vi "Command & Ack - Destroy Endpoints.vi"(8 "error in (no error)":errorcluster, 11 "SV B-M (Target) in":refnum<class "SV B-M (Target).lvclass">) -> (0 "error out":errorcluster, 3 "SV B-M (Target) out":refnum<class "SV B-M (Target).lvclass">)   [LabVIEW 2015, in "SV B-M (Target).lvclass"]
uses:
  SV B-M (Target).lvclass
  SV B-M (Target).lvclass/SV B-M (Target).ctl
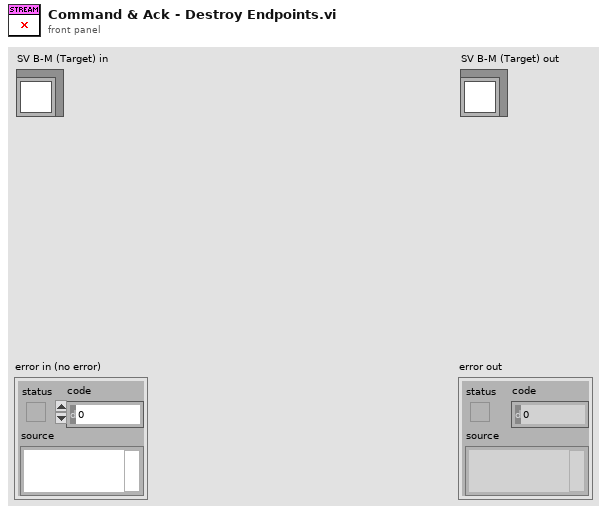
[diagram p1: front panel]
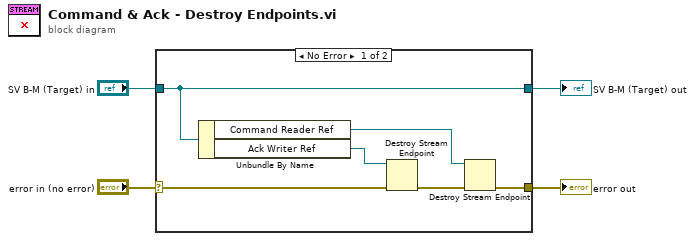
[diagram p0: block diagram]
diagram:
  n1 = case shown="No Error" "error in (no error)" {
    selector: "error in (no error)" -> [w8 w12]
    tunnel: [w5 w12] -> w3
    tunnel: [w10 w11] -> w1
    tunnel: "SV B-M (Target) in" -> [w10 w11]
    frame No Error {
      n2 = Unbundle By Name(w10) -> ("Command Reader Ref"=w6:refnum<k21>, "Ack Writer Ref"=w9:refnum<k21>)
      n3 = Destroy Stream Endpoint(8:w8, 11:w9) -> (0:w7:errorcluster)
      n4 = Destroy Stream Endpoint(8:w7, 11:w6) -> (0:w5:errorcluster)
    }
    frame Error {
    }
  }
  "error out" <- w3
  "SV B-M (Target) out" <- w1
